vi "Conditional Auto-Indexing Tunnel (I32)__ogtk.vi"(5 "Array in":i32[](array[numeric]), 6 "Elements to keep":bool[](array[boolean])) -> (1 "Filtered Array out":i32[](array[numeric]))   [LabVIEW 2011]
doc: "This polymorphic VI filters <B>Array In</B> by keeping only those elements where corresponding elements in <B>Elements to keep</B> are TRUE."
panel:
  # "Conditional Auto-Indexing Tunnel.vi\n\nA VI that simulates a conditional Auto-Indexing tunnel.\n\nPlease visit http://www.OpenG.org to learn about the\nOpen Source LabVIEW software movement.\n\nNOTICE -- YOU MUST LEAVE THIS NOTICE IN PLACE.  PER THE TERMS OF THE LICENSE BELOW, YOU MAY SUBLICENSE THIS SOFTWARE \nIN ANY WAY THAT DOES NOT CONFLICT WITH THIS LICENSE.\n\n### BSD License (http://www.opensource.org/licenses/bsd-license.php) Begin ###\n \nCopyright (c) 2002, Jim Kring <jim@jimkring.com>\n\nAll rights reserved.\n\nRedistribution and use in source and binary forms, with or without modification, are permitted provided that the following conditions are met:\n\n    * Redistributions of source code must retain the above copyright notice, this list of conditions and the following disclaimer.\n    * Redistributions in binary form must reproduce the above copyright notice, this list of conditions and the following disclaimer in the \n       documentation and/or other materials provided with the distribution.\n    * Neither the name of SciWare, James Kring, Inc., nor the names of its contributors may be used to endorse or promote products derived \n       from this software without specific prior written permission.\n\nTHIS SOFTWARE IS PROVIDED BY THE COPYRIGHT HOLDERS AND CONTRIBUTORS \"AS IS\" AND ANY EXPRESS OR IMPLIED WARRANTIES, \nINCLUDING, BUT NOT LIMITED TO, THE IMPLIED WARRANTIES OF MERCHANTABILITY AND FITNESS FOR A PARTICULAR PURPOSE ARE \nDISCLAIMED. IN NO EVENT SHALL THE COPYRIGHT OWNER OR CONTRIBUTORS BE LIABLE FOR ANY DIRECT, INDIRECT, INCIDENTAL,\n SPECIAL, EXEMPLARY, OR CONSEQUENTIAL DAMAGES (INCLUDING, BUT NOT LIMITED TO, PROCUREMENT OF SUBSTITUTE GOODS OR \nSERVICES; LOSS OF USE, DATA, OR PROFITS; OR BUSINESS INTERRUPTION) HOWEVER CAUSED AND ON ANY THEORY OF LIABILITY, \nWHETHER IN CONTRACT, STRICT LIABILITY, OR TORT (INCLUDING NEGLIGENCE OR OTHERWISE) ARISING IN ANY WAY OUT OF THE USE \nOF THIS SOFTWARE, EVEN IF ADVISED OF THE POSSIBILITY OF SUCH DAMAGE.\n\n### BSD License End ###"
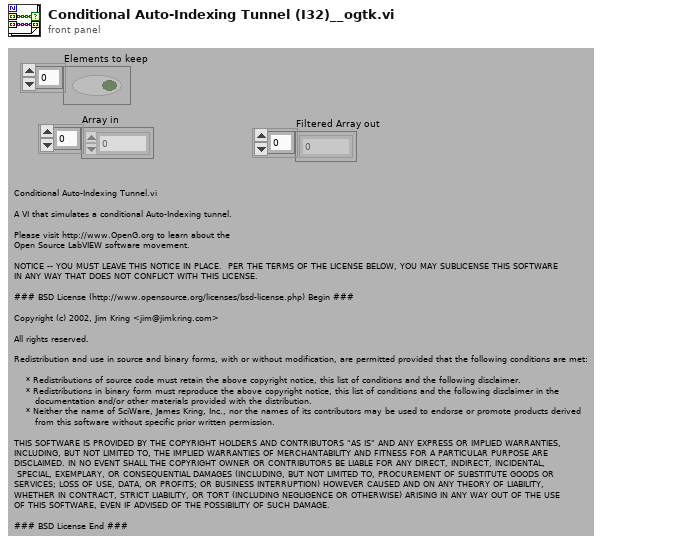
[diagram p1: front panel]
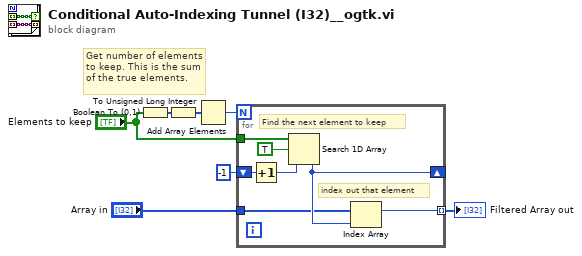
[diagram p0: block diagram]
diagram:
  # "Get number of elements to keep. This is the sum of the true elements."
  n1 = Boolean To (0,1)(Boolean="Elements to keep") -> (0, 1=w3:i16[])
  n2 = To Unsigned Long Integer(number=w3) -> (unsigned 32bit integer=w1:u32[])
  n3 = Add Array Elements(numeric array=w1) -> (sum=w4:u32)
  n4 = for {
    N: w4 -> [_]
    tunnel: "Array in" -> [w10]
    tunnel: "Elements to keep" -> [w14]
    shift-right: [w11] -> _
    shift-left: -1 ("start index (0)") -> [w12]
    tunnel: [w9] -> w7 mode=indexing
    # "index out that element"
    # "Find the next element to keep"
    n5 = Increment(x=w12) -> (x+1=w8:i32)
    n6 = Search 1D Array(1D array=w14, element=TRUE, start index (0)=w8) -> (index of element=w11:i32)
    n7 = Index Array(array=w10, index=w11) -> (element=w9:i32)
  }
  "Filtered Array out" <- w7
